vi "Update Count.vi"(8 "error in (no error)":errorcluster, 10 "Count":dbl, 11 "Chef UI Logic in":refnum<class "Chef UI Logic.lvclass">) -> (0 "error out":errorcluster, 3 "Chef UI Logic out":refnum<class "Chef UI Logic.lvclass">)   [LabVIEW 2024, in "Chef UI Logic.lvlib" / "Chef UI Logic.lvclass"]
uses:
  Chef UI Logic.lvclass
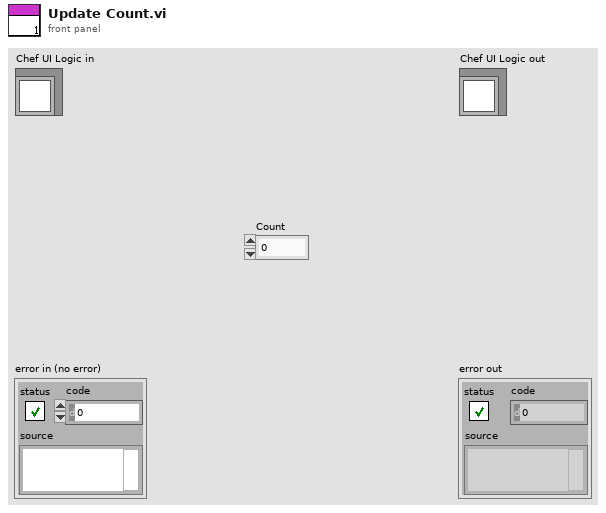
[diagram p1: front panel]
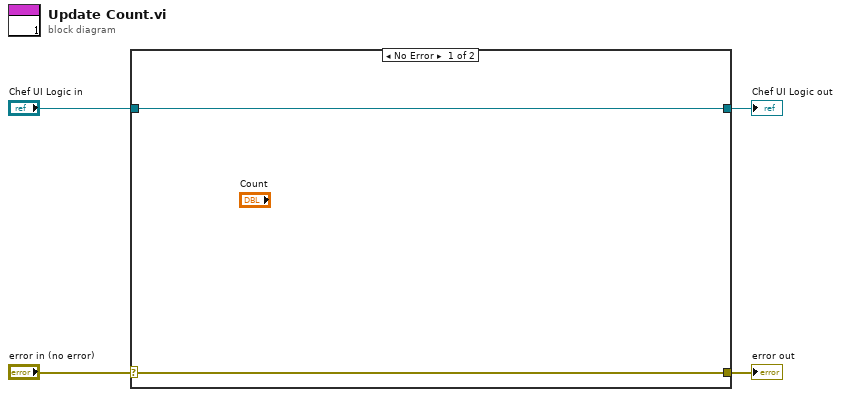
[diagram p0: block diagram]
diagram:
  n1 = case shown="No Error" "error in (no error)" {
    selector: "error in (no error)" -> [w5 w8]
    tunnel: [w5 w8] -> w3
    tunnel: [w6 w7] -> w1
    tunnel: "Chef UI Logic in" -> [w6 w7]
    frame No Error {
    }
    frame Error {
    }
  }
  "error out" <- w3
  "Chef UI Logic out" <- w1
